vi "Actor Core.vi"(8 "error in":errorcluster, 11 "Central Control in":refnum<class "Central Control.lvclass">) -> (0 "error out":errorcluster, 3 "Actor out":refnum<class "Actor.lvclass">)   [LabVIEW 2021, in "Central Control.lvlib" / "Central Control.lvclass"]
doc: "(<B>Filename</B>: Actor Framework.lvlib:Actor.lvclass:Actor Core.vi)\n\nReceives messages to the actor, reacts to them, and initiates any error handling that may shut the actor down.\n\nDescendant classes may override this VI to append parallel tasks for the actor to complete while it handles messages. Overrides use the Call Parent Class Method node."
uses:
  Central Control.lvclass
  C:/Program Files (x86)/National Instruments/LabVIEW 2021/vi.lib/ActorFramework/Actor/Actor.lvclass
  <vilib>/ActorFramework/Actor/Actor.lvclass
  Heating Control/Heating Control/Heating Control.lvclass
  Light Control/Light Control/Light Control.lvclass
  Central Control.lvclass/Central Control.ctl
  <vilib>/ActorFramework/Actor/Actor.lvclass/Actor.ctl
  <vilib>/ActorFramework/Message Enqueuer/Message Enqueuer.lvclass/Message Enqueuer.ctl
  Light Control/Light Control/Room List.ctl
  Light Control/Light Control Messages/Set Room Lamp State Msg/Set Room Lamp State Msg.lvclass/Set Room Lamp State Msg.ctl
  Heating Control/Heating Control Messages/Set Temperature Msg/Set Temperature Msg.lvclass/Set Temperature Msg.ctl
  <vilib>/ActorFramework/Message Enqueuer/Init from Existing Queue.vi
  <vilib>/ActorFramework/Message Enqueuer/Enqueue.vi
  <vilib>/ActorFramework/Stop Msg/Stop Msg.lvclass
  C:/Program Files (x86)/National Instruments/LabVIEW 2021/vi.lib/ActorFramework/Message/Message.lvclass
  Light Control/Light Control Messages/Set Room Lamp State Msg/Set Room Lamp State Msg.lvclass
  Heating Control/Heating Control Messages/Set Temperature Msg/Set Temperature Msg.lvclass
  <vilib>/ActorFramework/Message Priority Queue/Priority Enqueue.vi
  <vilib>/ActorFramework/Message Enqueuer/Message Enqueuer.lvclass
panel:
  in  "Set Temp":bool
  in  "Set Central Temperature(C)":dbl
  out "Set Point Value":dbl(knob) caption="Gauge" scale=0.0..50.0
  in  "Room-2":bool
  in  "Room-1":bool
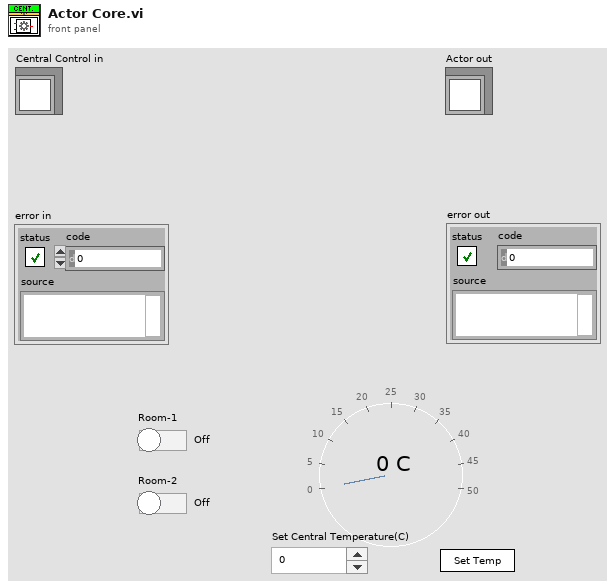
[diagram p1: front panel]
types:
  T1 = typedef "Light Control.lvlib/Light Control.lvclass/Room List.ctl" = enum16{"Room1", "Room2"}
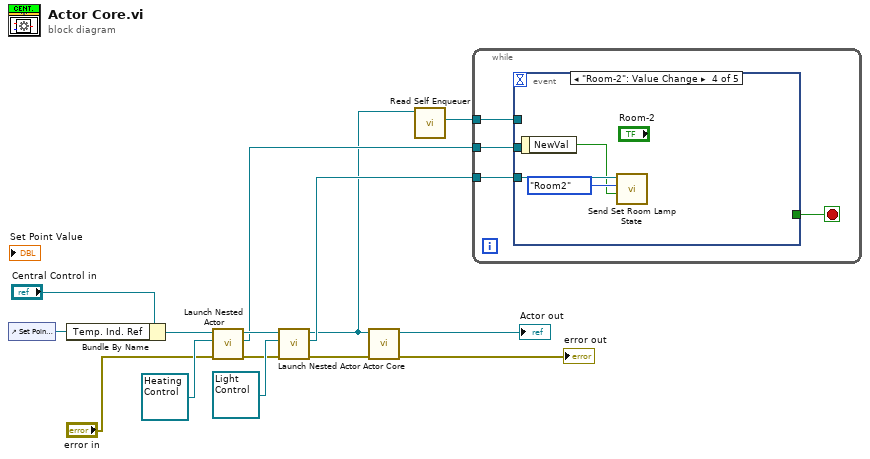
[diagram p0: block diagram]
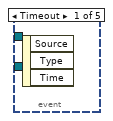
[diagram p2: hidden frame]
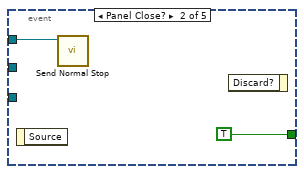
[diagram p3: hidden frame]
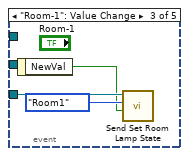
[diagram p4: hidden frame]
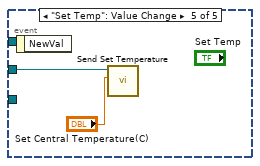
[diagram p5: hidden frame]
diagram:
  n1 = control-ref of="Set Point Value"() -> (w13:refnum<vi>)
  n2 = Bundle By Name(cluster="Central Control in", "Temp. Ind. Ref"=w13) -> (w12:refnum<class "Central Control.lvclass">)
  n3 = call <vilib>:"Launch Nested Actor.vi"("error in (no error)"="error in", "Nested Actor"=refnum<class "Heating Control.lvclass"> refnum ("Heating Control.lvlib:Heating Control.lvclass"), "Caller Actor in"=w12) -> ("error out"=w7:errorcluster, "Nested Actor's Enqueuer"=w5:refnum<class "Message Enqueuer.lvclass">, "Caller Actor out"=w10:refnum<class "Central Control.lvclass">)  [unwired: 6 in]
  n4 = call <vilib>:"Launch Nested Actor.vi"("error in (no error)"=w7, "Nested Actor"=refnum<class "Light Control.lvclass"> refnum ("Light Control.lvlib:Light Control.lvclass"), "Caller Actor in"=w10) -> ("error out"=w6:errorcluster, "Nested Actor's Enqueuer"=w4:refnum<class "Message Enqueuer.lvclass">, "Caller Actor out"=w1:refnum<class "Central Control.lvclass">)  [unwired: 6 in]
  n5 = call-parent "Actor Core.vi"("error in"=w6, "Actor in"=w1) -> ("error out"=→"error out":errorcluster, "Actor out"=→"Actor out":refnum<class "Actor.lvclass">)  [unwired: 8 in]
  n6 = call <vilib>:"Read Self Enqueuer.vi"("Actor"=w1) -> ("Self Enqueuer"=w2:refnum<class "Message Enqueuer.lvclass">)  [unwired: 10 in]
  n7 = while {
    tunnel: w5 -> [w18]
    tunnel: w4 -> [w19]
    tunnel: w2 -> [w17]
    stop <- w16 stop-if-true
    n8 = event shown="[3] \"Room-2\": Value Change" {
      selector: _ -> [_ _ _ _ _]
      dyn-events: _ -> [_ _ _ _ _]
      timeout: _ -> [_ _ _ _ _]
      tunnel: w19 -> [_ _ w24 w27 _]
      tunnel: w18 -> [_ _ _ _ w29]
      tunnel: w17 -> [_ w21 _ _ _]
      tunnel: [_ TRUE _ _ _] -> w16
      event Timeout {
        n9 = event-data() -> ()  [unwired: 1 in, 3 out]
      }
      event Panel Close? {
        n10 = event-data() -> ()  [unwired: 1 in, 1 out]
        n11 = call <vilib>:"Send Normal Stop.vi"("Message Enqueuer"=w21) -> ()  [unwired: 10 in, 1 out]
        n12 = event-data() -> ()  [unwired: 2 in, 1 out]
      }
      event "Room-1": Value Change {
        n13 = event-data() -> ("NewVal"=w22:bool)  [unwired: 1 in]
        n14 = call "Send Set Room Lamp State.vi"("Value"=w22, "Room List"=Room_List."Room1", "Message Enqueuer in"=w24) -> ()  [unwired: 7 in, 2 out]
      }
      event "Room-2": Value Change {
        n15 = event-data() -> ("NewVal"=w25:bool)  [unwired: 1 in]
        n16 = call "Send Set Room Lamp State.vi"("Value"=w25, "Room List"=Room_List."Room2", "Message Enqueuer in"=w27) -> ()  [unwired: 7 in, 2 out]
      }
      event "Set Temp": Value Change {
        n17 = event-data() -> ()  [unwired: 1 in, 1 out]
        n18 = call "Send Set Temperature.vi"("Set Point(C)"="Set Central Temperature(C)", "Message Enqueuer in"=w29) -> ()  [unwired: 8 in, 2 out]
      }
    }
  }
